vi "Get SMO Port.vi"(8 "error in (no error)":errorcluster, 11 "instrument.PPMS in":refnum<class "instrument.PPMS-W-1.lvclass">) -> (0 "error out":errorcluster, 2 "Port":u16, 3 "instrument.PPMS out":refnum<class "instrument.PPMS-W-1.lvclass">)   [LabVIEW 2019, in "instrument.PPMS-W-1.lvclass"]
uses:
  instrument.PPMS-W-1.lvclass
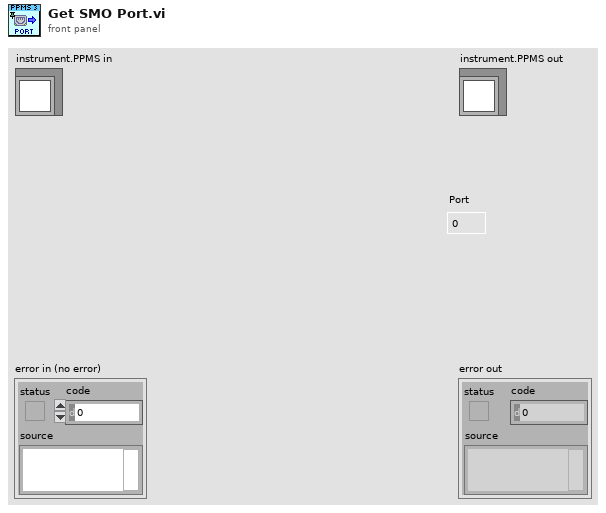
[diagram p1: front panel]
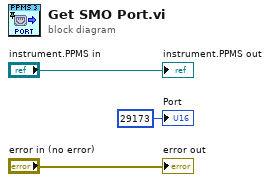
[diagram p0: block diagram]
diagram:
  "error out" <- "error in (no error)"
  "instrument.PPMS out" <- "instrument.PPMS in"
  "Port" <- u16 29173 ("Port")
